vi "Single run tests.vi"(8 "error in (no error)":errorcluster, 10 "Measurement settings":T1={"Source Mode "=1, "Source Level"=0.0001, "Source Limit"=10.0, "Measure Function"=0, "Remote sense"=FALSE, "Clear buffer?"=FALSE, "Beep"=FALSE, "High Capacity"=FALSE, "Terminals"=0, "PLCs"=0.5} {"Measure Function" items=["Volts", "Current", "Auto Resistance", "Manual Resistance", "Digitize Voltage", "Digitize Current"]; "Source Mode" items=["Front", "Rear"]; "Terminals" items=["Front", "Rear"]}) -> (0 "error out":errorcluster, 3 "SMU status out":T2)   [LabVIEW 2017, in "Source meter.lvlib"]
uses:
  Source meter.lvlib
  ctls/SMU status.ctl
  ctls/SMU settings.ctl
  <instrlib>/Keithley 2450/Keithley 2450.lvlib
panel:
  in  "VISA resource name":refnum<visa-resource-name>
  in  "error in (no error) 2":errorcluster
  out "Data out":string
  out "x-y":u32
  out "time":u32
  in  "VISA name":refnum<visa-resource-name>
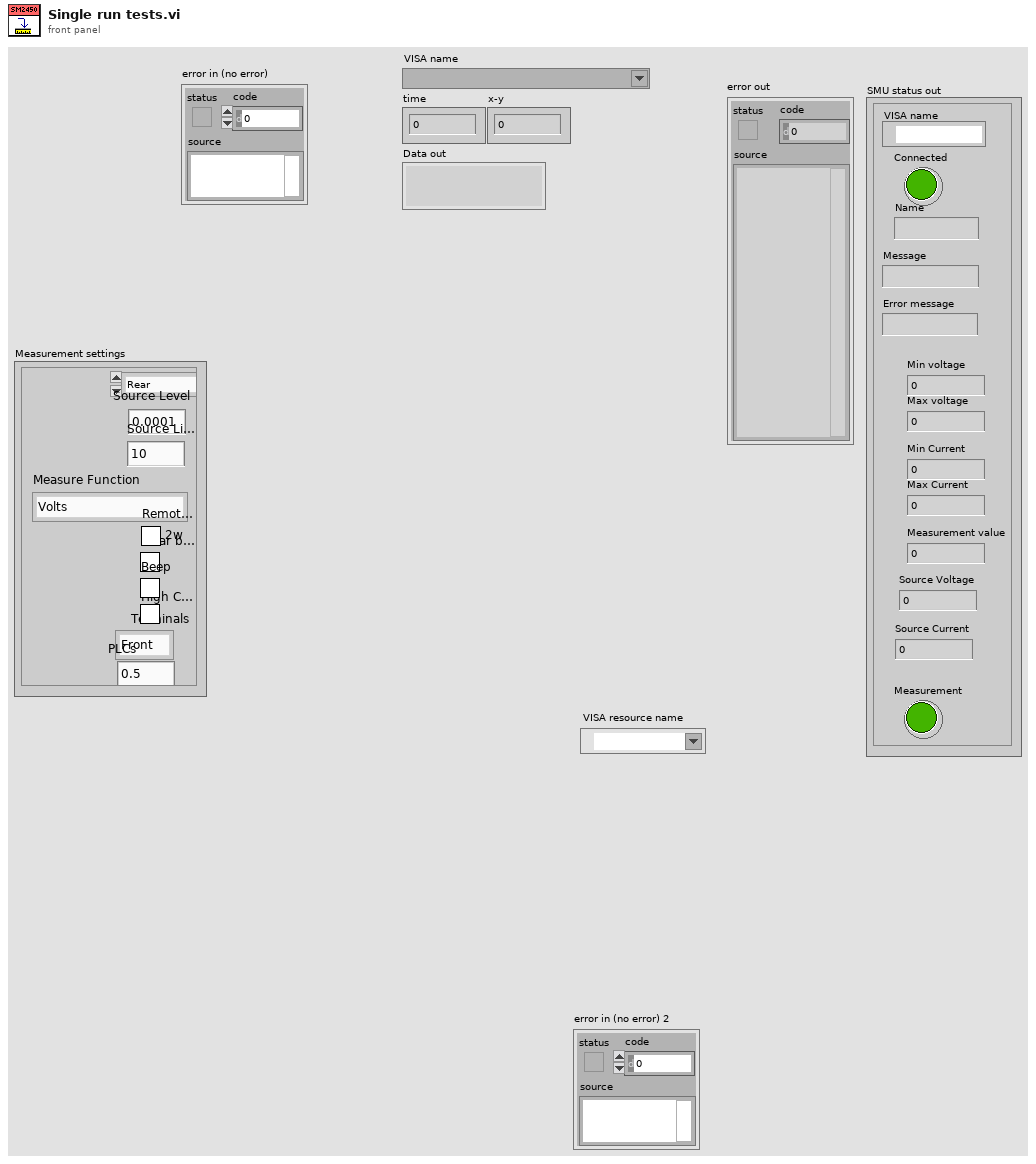
[diagram p1: front panel]
types:
  T1 = typedef "SMU settings.ctl" = cluster{"Source Mode ":u16, "Source Level":dbl, "Source Limit":dbl, "Measure Function":u16, "Remote sense":bool, "Clear buffer?":bool, "Beep":bool, "High Capacity":bool, "Terminals":u16, "PLCs":dbl}
  T2 = typedef "Source meter.lvlib/SMU status.ctl" = cluster{"VISA name":refnum<visa-resource-name>, "Connected":bool, "Name":string, "Message":string, "Error message":string, "Min voltage":dbl, "Max voltage":dbl, "Min Current":dbl, "Max Current":dbl, "Measurement value":dbl, "Source Voltage":dbl, "Measurement":bool, "Source Current":dbl}
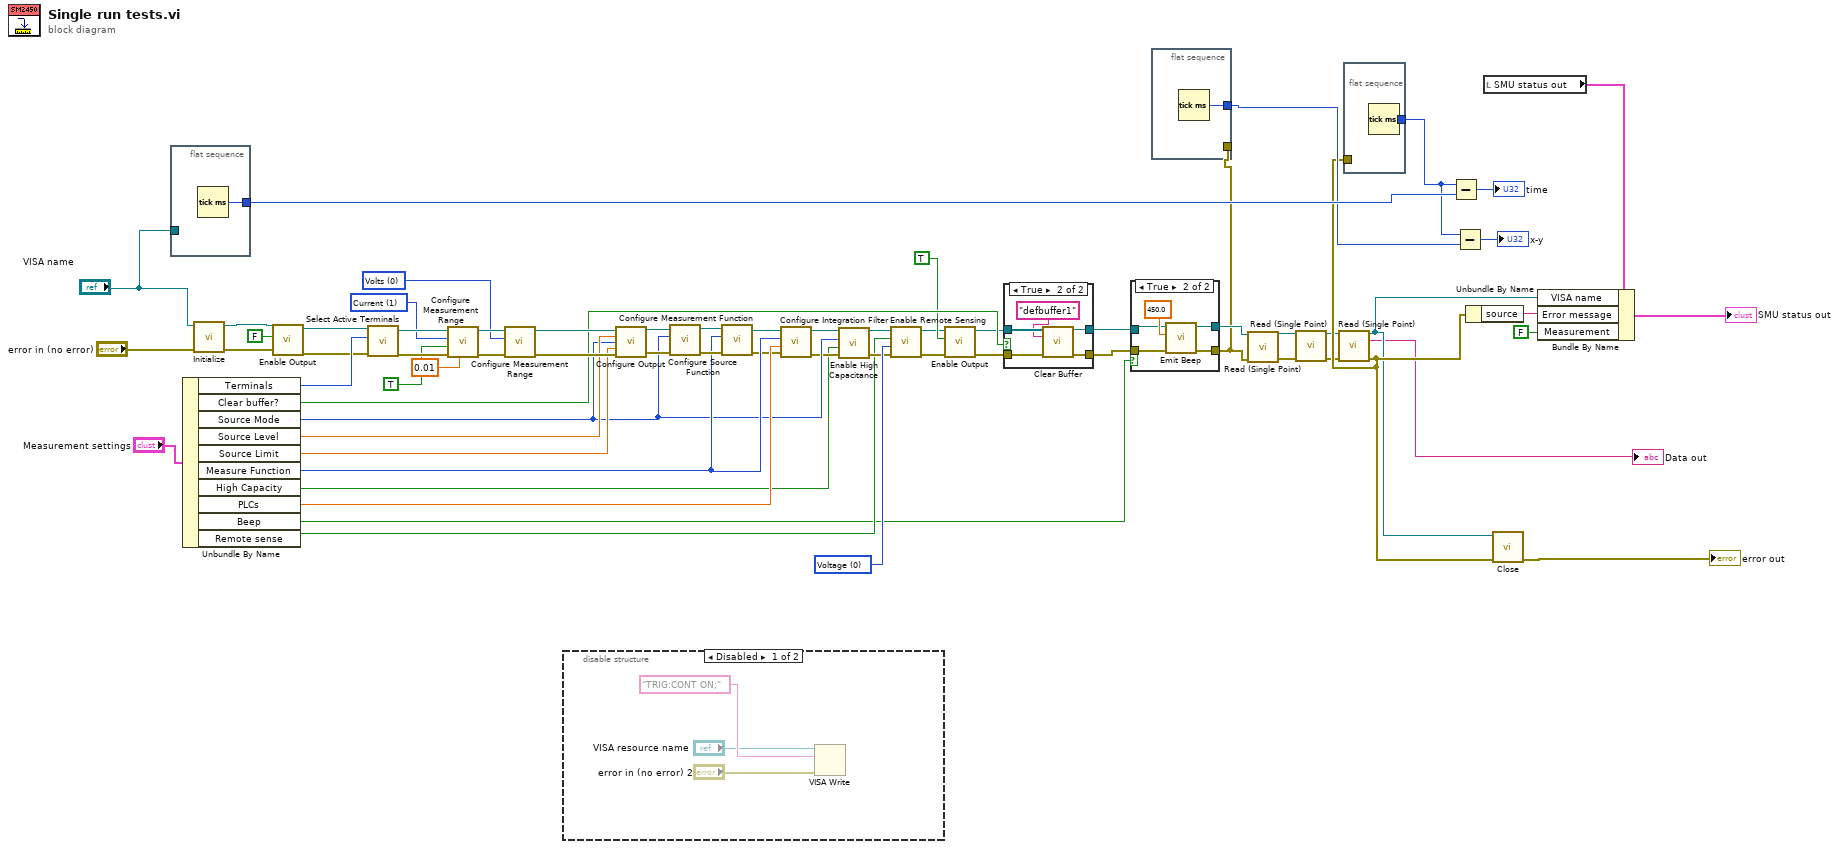
[diagram p0: block diagram]
diagram:
  w32 = u16 0 items=["Voltage", "Current", "Resistance", "Digitize Voltage", "Digitize Current"] ("Function (0:Voltage)")
  w57 = u16 0 items=["Volts", "Current", "Resistance"] ("Function (0: Volts)")
  w60 = u16 1 items=["Volts", "Current", "Resistance"] ("Function (0: Volts)")
  n1 = flat-sequence {
    tunnel: "VISA name" -> [_]
    tunnel: [w66] -> w25
    frame #0 {
      n2 = Tick Count (ms)() -> (millisecond timer value=w66:u32)
    }
  }
  n3 = Unbundle By Name("Measurement settings") -> ("Terminals"=w55:u16, "Clear buffer?"=w44:bool, "Source Mode"=w39:u16, "Source Level"=w50:dbl, "Source Limit"=w49:dbl, "Measure Function"=w40:u16, "High Capacity"=w36:bool, "PLCs"=w41:dbl, "Beep"=w13:bool, "Remote sense"=w14:bool)
  n4 = call <instrlib>:"Initialize.vi"("error in (no error)"="error in (no error)", "VISA resource name"="VISA name") -> ("error out"=w31:errorcluster, "VISA resource name out"=w30:refnum<visa-resource-name>)  [unwired: 8 in]
  n5 = call <instrlib>:"Enable Output.vi"("error in (no error)"=w31, "Enable Output (T: Enable)"=FALSE, "VISA resource name"=w30) -> ("error out"=w11:errorcluster, "VISA resource name out"=w12:refnum<visa-resource-name>)  [unwired: 7 in]
  n6 = call <instrlib>:"Select Active Terminals.vi"("error in (no error)"=w11, "Active Terminals (0: Front)"=w55, "VISA resource name"=w12) -> ("error out"=w62:errorcluster, "VISA resource name out"=w63:refnum<visa-resource-name>)  [unwired: 7 in]
  n7 = call <instrlib>:"Configure Measurement Range.vi"("Manual Range (1.0)"=0.01, "error in (no error)"=w62, "Enable Auto Range (T:Enable)"=TRUE, "Function (0: Volts)"=w60, "VISA resource name"=w63) -> ("error out"=w59:errorcluster, "VISA resource name out"=w58:refnum<visa-resource-name>)  [unwired: 5 in]
  n8 = call <instrlib>:"Configure Measurement Range.vi"("error in (no error)"=w59, "Function (0: Volts)"=w57, "VISA resource name"=w58) -> ("error out"=w54:errorcluster, "VISA resource name out"=w53:refnum<visa-resource-name>)  [unwired: 7 in]
  n9 = disable-structure shown="Disabled" {
    frame Disabled {
      n10 = VISA Write(VISA resource name="VISA resource name", write buffer="TRIG:CONT ON;", error in (no error)="error in (no error) 2") -> ()  [unwired: 3 out]
    }
    frame Enabled {
    }
  }
  n11 = call <instrlib>:"Configure Output.vi"("VISA resource name"=w53, "Source Level (0)"=w50, "Source Mode  (0: Voltage)"=w39, "Source Limit Level (0.1)"=w49, "error in (no error)"=w54) -> ("VISA resource name out"=w51:refnum<visa-resource-name>, "error out"=w52:errorcluster)  [unwired: 9 in]
  n12 = call <instrlib>:"Configure Source Function.vi"("error in (no error)"=w52, "Function (0: Volts)"=w39, "VISA resource name"=w51) -> ("error out"=w47:errorcluster, "VISA resource name out"=w48:refnum<visa-resource-name>)  [unwired: 7 in]
  n13 = call <instrlib>:"Configure Measurement Function.vi"("error in (no error)"=w47, "Function (0: Volts)"=w40, "VISA resource name"=w48) -> ("error out"=w34:errorcluster, "VISA resource name out"=w35:refnum<visa-resource-name>)  [unwired: 7 in]
  n14 = call <instrlib>:"Configure Integration Filter.vi"("error in (no error)"=w34, "Measurement Speed (1 PLC)"=w41, "Function (0: Volts)"=w40, "VISA resource name"=w35) -> ("error out"=w38:errorcluster, "VISA resource name out"=w37:refnum<visa-resource-name>)  [unwired: 6 in]
  n15 = call <instrlib>:"Enable High Capacitance.vi"("error in (no error)"=w38, "Enable High Capacitance (T:Enable)"=w36, "Function (0: Volts)"=w39, "VISA resource name"=w37) -> ("error out"=w20:errorcluster, "VISA resource name out"=w21:refnum<visa-resource-name>)  [unwired: 6 in]
  n16 = call <instrlib>:"Enable Remote Sensing.vi"("error in (no error)"=w20, "Function (0:Voltage)"=w32, "Enable Remote Sensing (T: Enable)"=w14, "VISA resource name"=w21) -> ("error out"=w19:errorcluster, "VISA resource name out"=w18:refnum<visa-resource-name>)  [unwired: 6 in]
  n17 = call <instrlib>:"Enable Output.vi"("error in (no error)"=w19, "Enable Output (T: Enable)"=TRUE, "VISA resource name"=w18) -> ("error out"=w22:errorcluster, "VISA resource name out"=w23:refnum<visa-resource-name>)  [unwired: 7 in]
  n18 = case shown="True" w44 {
    tunnel: [w71 w76] -> w43
    tunnel: [w70 w75] -> w42
    tunnel: w22 -> [w71 w74]
    tunnel: w23 -> [w70 w73]
    frame False {
    }
    frame True {
      n19 = call <instrlib>:"Clear Buffer.vi"("VISA resource name"=w73, "Buffer Name (defbuffer1)"="defbuffer1", "error in (no error)"=w74) -> ("VISA resource name out"=w75:refnum<visa-resource-name>, "error out"=w76:errorcluster)  [unwired: 11 in]
    }
  }
  n20 = case shown="True" w13 {
    tunnel: [w77 w83] -> w2
    tunnel: [w78 w82] -> w3
    tunnel: w43 -> [w77 w80]
    tunnel: w42 -> [w78 w79]
    frame False {
    }
    frame True {
      n21 = call <instrlib>:"Emit Beep.vi"("error in (no error)"=w80, "Beep Frequency (300)"=450.0, "VISA resource name"=w79) -> ("error out"=w83:errorcluster, "VISA resource name out"=w82:refnum<visa-resource-name>)  [unwired: 7 in]
    }
  }
  n22 = flat-sequence {
    tunnel: [w84] -> w16
    tunnel: w2 -> [_]
    frame #0 {
      n23 = Tick Count (ms)() -> (millisecond timer value=w84:u32)
    }
  }
  n24 = call <instrlib>:"Read (Single Point).vi"("VISA resource name"=w3, "error in (no error)"=w2) -> ("VISA resource name out"=w4:refnum<visa-resource-name>, "error out"=w6:errorcluster)  [unwired: 11 in, 1 out]
  n25 = call <instrlib>:"Read (Single Point).vi"("VISA resource name"=w4, "error in (no error)"=w6) -> ("VISA resource name out"=w8:refnum<visa-resource-name>, "error out"=w7:errorcluster)  [unwired: 11 in, 1 out]
  n26 = call <instrlib>:"Read (Single Point).vi"("VISA resource name"=w8, "error in (no error)"=w7) -> ("VISA resource name out"=w5:refnum<visa-resource-name>, "Data out"=→"Data out":string, "error out"=w9:errorcluster)  [unwired: 11 in]
  n27 = flat-sequence {
    tunnel: [w85] -> w17
    tunnel: w9 -> [_]
    frame #0 {
      n28 = Tick Count (ms)() -> (millisecond timer value=w85:u32)
    }
  }
  n29 = Subtract(x=w17, y=w25) -> (x-y=→"time":u32)
  n30 = Subtract(x=w17, y=w16) -> (x-y=→"x-y":u32)
  n31 = Unbundle By Name(w9) -> ("source"=w46:string)
  n32 = local read "SMU status out"() -> (w27:T2)
  n33 = call <instrlib>:"Close.vi"("error in (no error)"=w9, "VISA resource name"=w5) -> ("error out"=→"error out":errorcluster)  [unwired: 9 in]
  n34 = Bundle By Name(cluster=w27, "VISA name"=w5, "Error message"=w46, "Measurement"=FALSE) -> (→"SMU status out":T2)
